vi "Evaluate Captured Waveforms 1.vi"(8 "error in":errorcluster, 11 "Captured Waveforms":T1(graph)) -> (0 "error out":errorcluster, 3 "Response Passed?":bool)   [LabVIEW 2025]
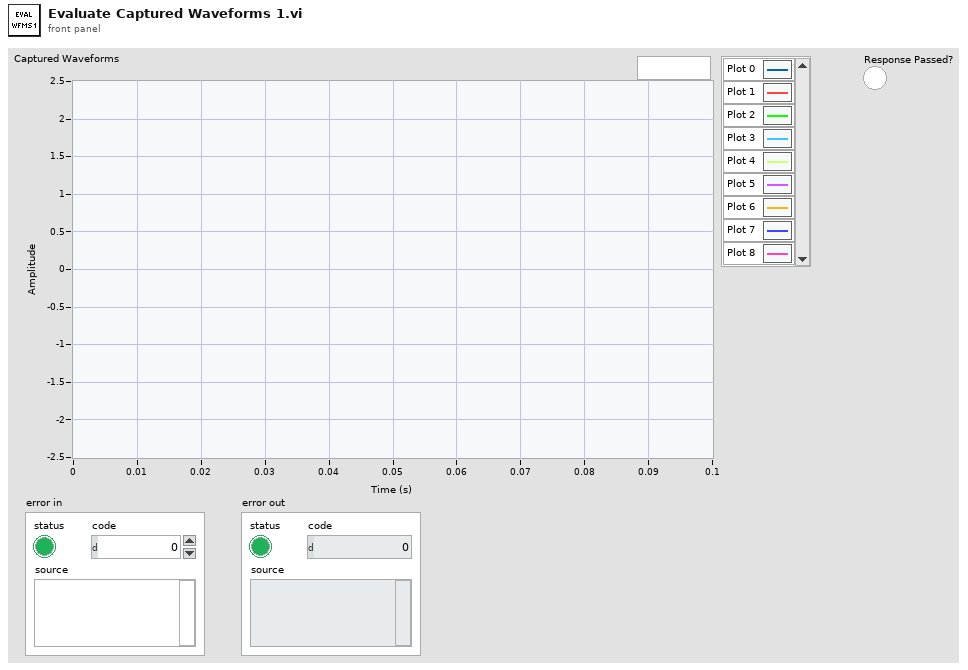
[diagram p1: front panel]
types:
  T1 = cluster{"relativeInitialX":dbl, "xIncrement":dbl, "wfm":dbl[]}[]
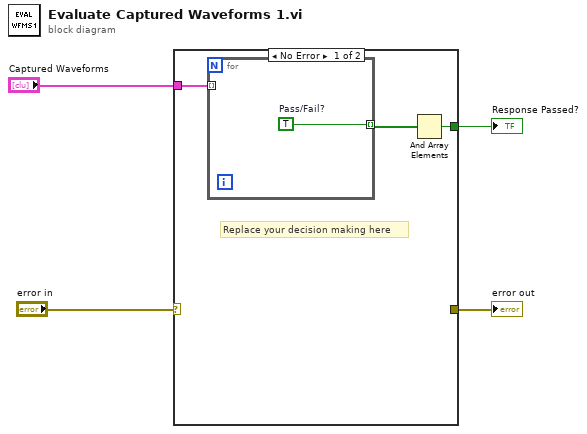
[diagram p0: block diagram]
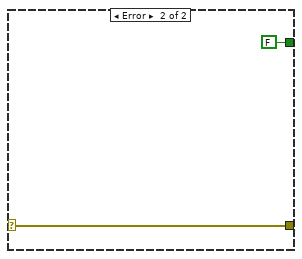
[diagram p2: hidden frame]
diagram:
  n1 = case shown="No Error" "error in" {
    selector: "error in" -> [_ w10]
    tunnel: [w7 FALSE] -> w4
    tunnel: "Captured Waveforms" -> [w5 _]
    tunnel: [_ w10] -> w1
    frame No Error {
      # "Replace your decision making here"
      n2 = for {
        tunnel: w5 -> [_] mode=indexing
        tunnel: [w8] -> w6 mode=indexing
        w8 = TRUE  # Pass/Fail?
      }
      n3 = And Array Elements(Boolean array=w6) -> (logical AND=w7:bool)
    }
    frame Error {
    }
  }
  "Response Passed?" <- w4
  "error out" <- w1
